vi "Get Array Indexing Settings.vi"(8 "error in (no error)":errorcluster, 11 "CConfig Variant Accessor in":refnum<class "CConfig Variant Accessor.lvclass">) -> (0 "error out":errorcluster, 1 "Array indexing":bool, 2 "Index":i32, 3 "CConfig Variant Accessor out":refnum<class "CConfig Variant Accessor.lvclass">)   [LabVIEW 2013, in "CConfig Variant Accessor.lvclass"]
doc: "Copyright 2018, Carya Automatisering, Wiebe Walstra."
uses:
  CConfig Variant Accessor.lvclass
  CConfig Variant Accessor.lvclass/CConfig Variant Accessor.ctl
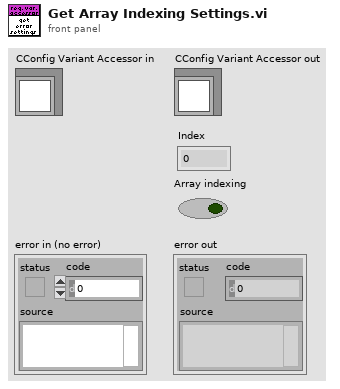
[diagram p1: front panel]
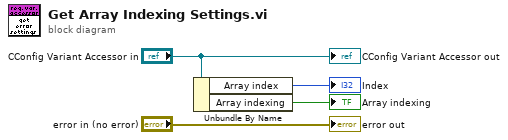
[diagram p0: block diagram]
diagram:
  n1 = Unbundle By Name("CConfig Variant Accessor in") -> ("Array index"=→"Index":i32, "Array indexing"=→"Array indexing":bool)
  "error out" <- "error in (no error)"
  "CConfig Variant Accessor out" <- "CConfig Variant Accessor in"
